vi "Write Pointer Size.vi"(9 "offset":i32, 10 "error in":errorcluster, 11 "Pointer in":refnum<class "Pointer.lvclass">) -> (1 "new offset":i32, 2 "error out":errorcluster, 3 "Pointer out":refnum<class "Pointer.lvclass">)   [LabVIEW 2017, in "Memory Manager.lvlib" / "Pointer.lvclass"]
uses:
  Pointer.lvclass
  Pointer.lvclass/Pointer.ctl
  VIs/VIs for Poly/Write U64 into Source.vi
  Deterministic Error Builder.lvlib
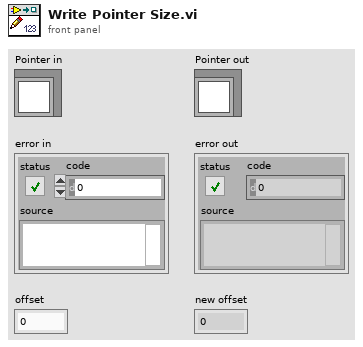
[diagram p1: front panel]
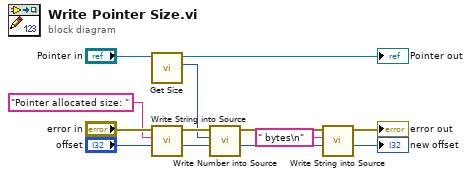
[diagram p0: block diagram]
diagram:
  n1 = call "Get Size.vi"("Pointer in"="Pointer in") -> ("size"=w7:u64, "Pointer out"=→"Pointer out":refnum<class "Pointer.lvclass">)  [unwired: 9 in]
  n2 = call "Write String into Source.vi"("offset"="offset", "string"="Pointer allocated size: ", "error in"="error in") -> ("new offset"=w12:i32, "error out"=w13:errorcluster)  [unwired: 7 in]
  n3 = call-poly "Write Number into Source.vi"("offset"=w12, "value"=w7, "error in"=w13) -> ("new offset"=w5:i32, "error out"=w6:errorcluster)  [unwired: 7 in]
  n4 = call "Write String into Source.vi"("offset"=w5, "string"=" bytes\n", "error in"=w6) -> ("new offset"=→"new offset":i32, "error out"=→"error out":errorcluster)  [unwired: 7 in]
